vi "fgv_캐패시터부하_config.vi"(7 "cmd":T2, 11 "캐패시터부하":T1) -> (3 "캐패시터부하 2":T1)   [LabVIEW 2019]
uses:
  _ctrl/rw.ctl
panel:
  # "고전압"
  # "충전기준"
  # "제어전압"
  # "고전압"
  # "충전기준"
  # "제어전압"
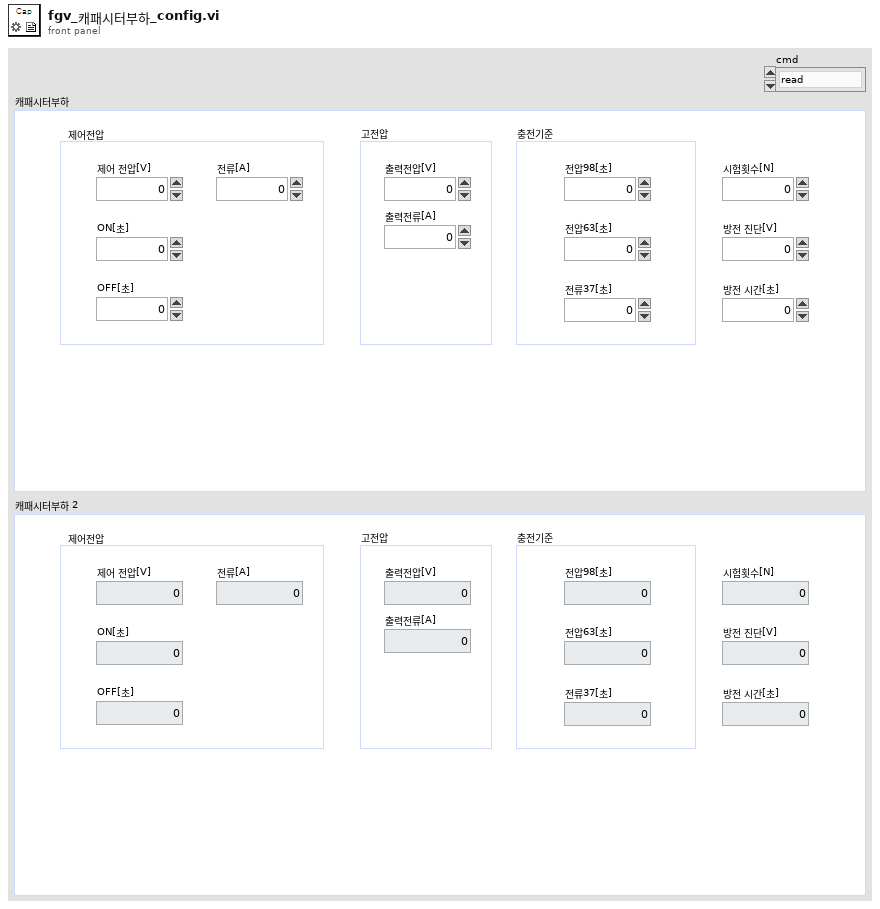
[diagram p1: front panel]
types:
  T1 = cluster{"제어 전압[V]":dbl, "출력전압[V]":dbl, "전류[A]":dbl, "출력전류[A]":dbl, "ON[초]":dbl, "OFF[초]":dbl, "시험횟수[N]":dbl, "방전 진단[V]":dbl, "전압98[초]":dbl, "전압63[초]":dbl, "전류37[초]":dbl, "방전 시간[초]":dbl}
  T2 = typedef "rw.ctl" = enum16{"read", "write"}
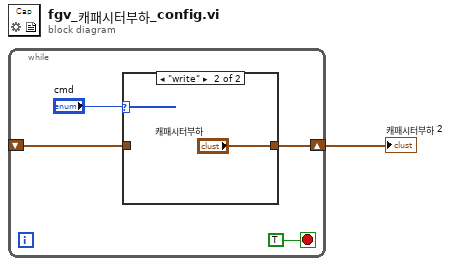
[diagram p0: block diagram]
diagram:
  n1 = while {
    shift-right: [w4] -> w1
    shift-left: _ -> [w3]
    stop <- TRUE stop-if-true
    n2 = case shown="\"write\"" "cmd" {
      tunnel: [w6 "캐패시터부하"] -> w4
      tunnel: w3 -> [w6 _]
      frame "read", Default {
      }
      frame "write" {
      }
    }
  }
  "캐패시터부하 2" <- w1
